vi "ICS425.vi"(0 "VISA resource name":refnum<visa-resource-name>="SETRA", 11 "Error In":errorcluster) -> (15 "Error Out":errorcluster)   [LabVIEW 2016]
panel:
  out "concatenated string":string
  in  "Commad":string
  out "Read Buffer":string
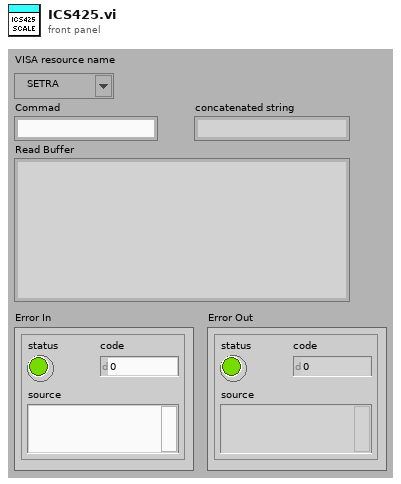
[diagram p1: front panel]
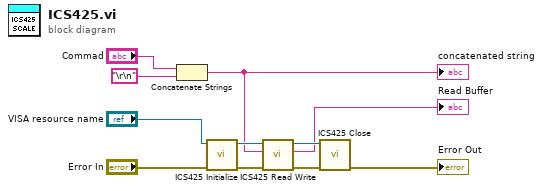
[diagram p0: block diagram]
diagram:
  n1 = Concatenate Strings("Commad", "\r\n") -> (w3:string)
  "concatenated string" <- w3
  n2 = call "ICS425 Initialize.vi"("Error In"="Error In", "VISA Refnum in"="VISA resource name") -> ("Error Out"=w8:errorcluster, "VISA Refnum out"=w9:refnum<visa-resource-name>)  [unwired: 8 in]
  n3 = call "ICS425 Read Write.vi"("Error In"=w8, "Cmd"=w3, "VISA (Input)"=w9) -> ("Error Out"=w6:errorcluster, "read buffer"=→"Read Buffer":string, "VISA Refnum (Output)"=w7:refnum<visa-resource-name>)  [unwired: 6 in]
  n4 = call "ICS425 Close.vi"("Error In"=w6, "VISA Refnum in"=w7) -> ("Error Out"=→"Error Out":errorcluster)  [unwired: 9 in]
